vi "set_tilt_stage (SubVI).vi"(2 "stop":bool, 3 "Tot Stage Arr":dbl[](array[numeric]), 4 "tilt stage config":T2) -> (0 "thetaZ error out":errorcluster, 1 "thetaY error out":errorcluster)   [LabVIEW 2016]
uses:
  C:/Users/UsphereLab/Documents/GitHub/Optlev/LabView Code/Tilt Stage/CmdLib.dll
  Tilt Stage/CmdLib.dll
panel:
  in  "Axis inputs 5":T1={"Relative Steps"=0, "Motor Number"=1, "Run?"=FALSE, "Filename"=path "position.lvm", "CmdLib In"=refnum, "Device Address In"=0, "DeviceKey In"=""}
  in  "Axis inputs 4":T1={"Relative Steps"=0, "Motor Number"=1, "Run?"=FALSE, "Filename"=path "position.lvm", "CmdLib In"=refnum, "Device Address In"=0, "DeviceKey In"=""}
  in  "B Inputs":T1={"Relative Steps"=0, "Motor Number"=1, "Run?"=FALSE, "Filename"=path "position.lvm", "CmdLib In"=refnum, "Device Address In"=0, "DeviceKey In"=""}
  in  "A inputs":T1={"Relative Steps"=0, "Motor Number"=1, "Run?"=FALSE, "Filename"=path "position.lvm", "CmdLib In"=refnum, "Device Address In"=0, "DeviceKey In"=""}
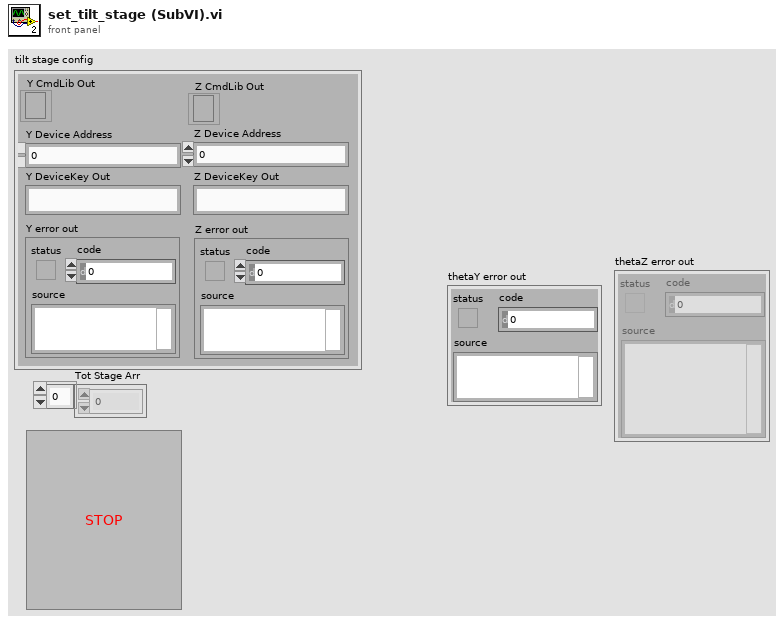
[diagram p1: front panel]
types:
  T1 = cluster{"Relative Steps":i32, "Motor Number":i32, "Run?":bool, "Filename":path, "CmdLib In":refnum<k24>, "Device Address In":i32, "DeviceKey In":string}
  T2 = cluster{"Y error out":errorcluster, "Y CmdLib Out":refnum<k24>, "Y Device Address":i32, "Y DeviceKey Out":string, "Z error out":errorcluster, "Z CmdLib Out":refnum<k24>, "Z Device Address":i32, "Z DeviceKey Out":string}
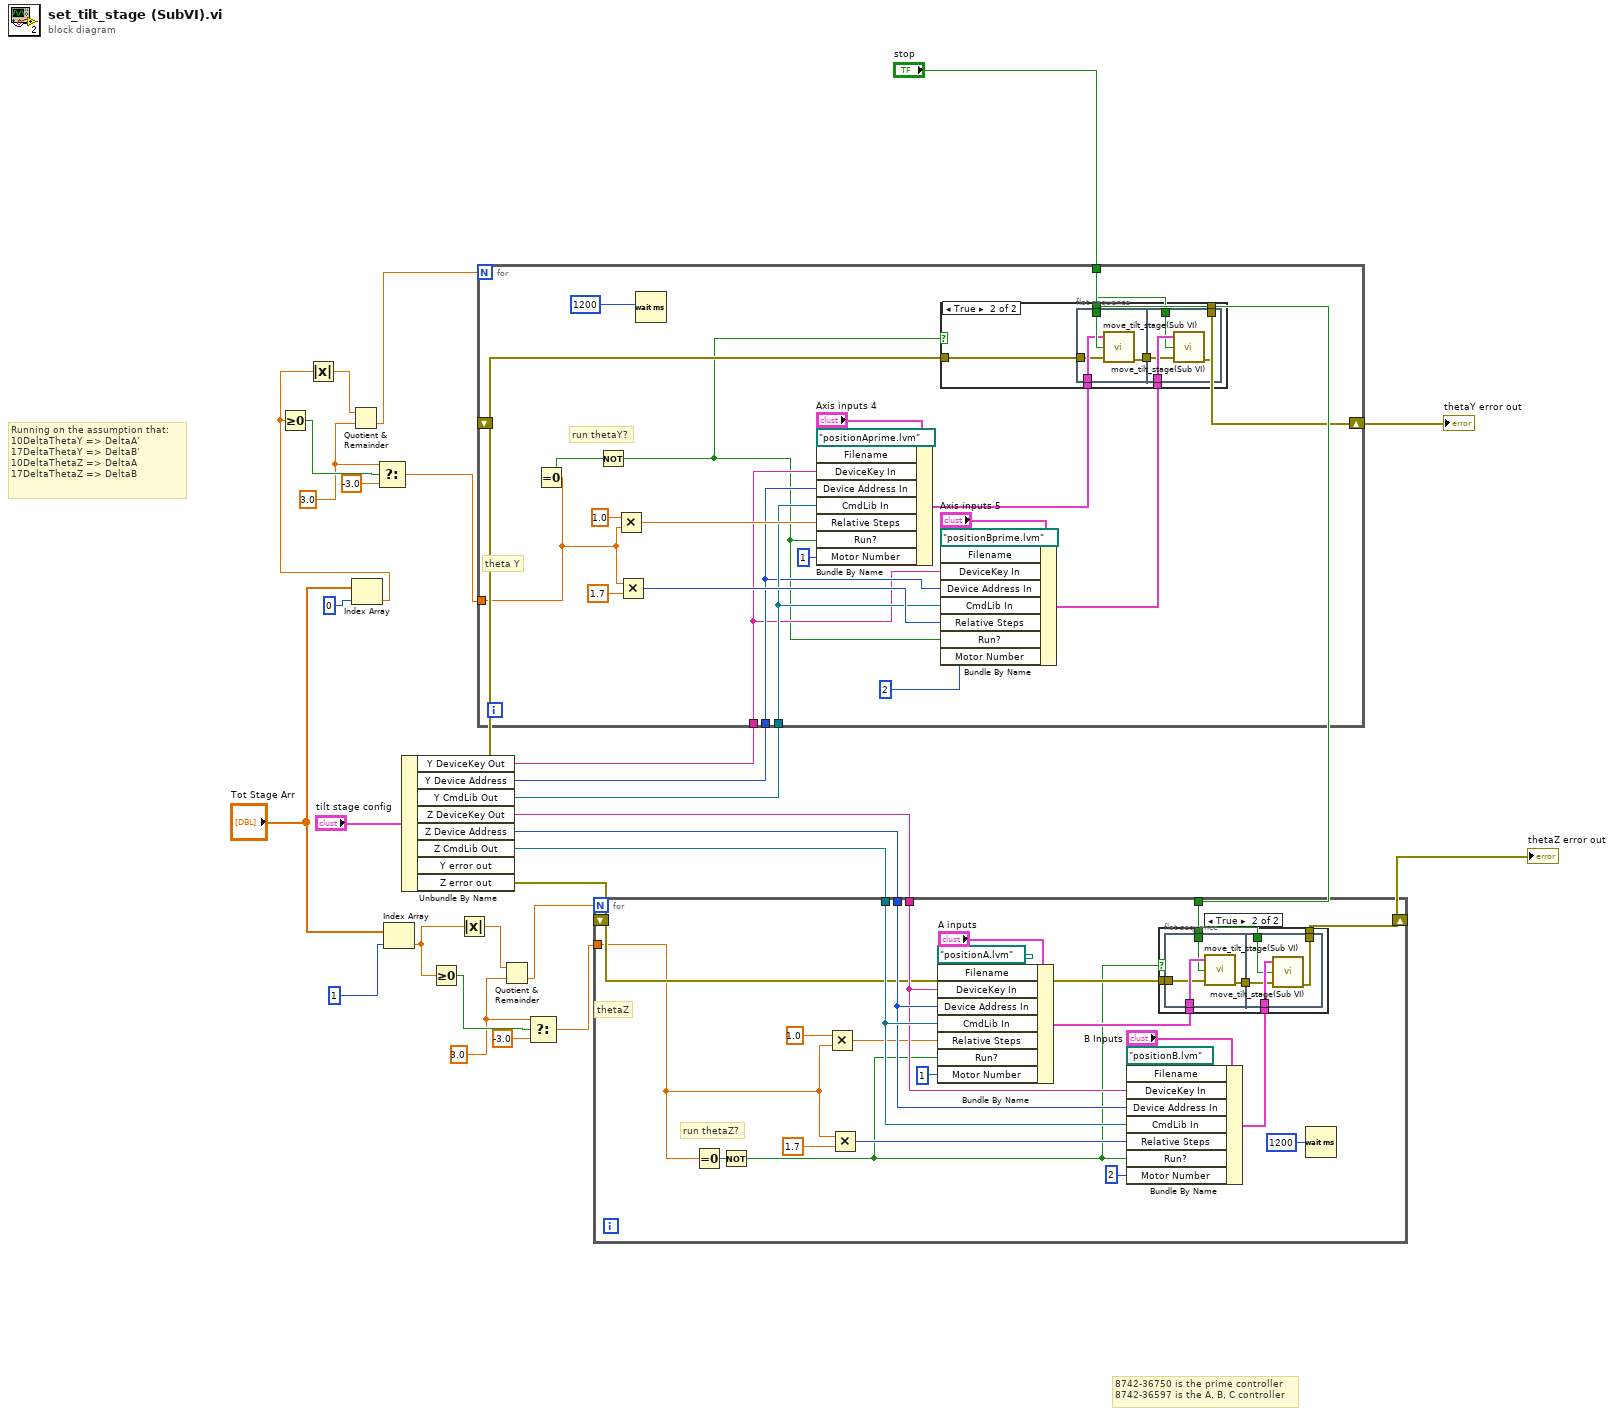
[diagram p0: block diagram]
diagram:
  w5 = 3.0 ("y")
  w10 = 3.0 ("y")
  # "Running on the assumption that:\n10DeltaThetaY => DeltaA'\n17DeltaThetaY => DeltaB'\n10DeltaThetaZ => DeltaA\n17DeltaThetaZ => DeltaB"
  # "8742-36750 is the prime controller\n8742-36597 is the A, B, C controller"
  n1 = Index Array(array="Tot Stage Arr", index=0 ("index (row)")) -> (element=w3:dbl)
  n2 = Greater Or Equal To 0?(x=w3) -> (x >= 0?=w6:bool)
  n3 = Absolute Value(x=w3) -> (abs(x)=w7:dbl)
  n4 = Quotient & Remainder(x=w7, y=w5) -> (floor(x/y)=w2:dbl)  [unwired: 1 out]
  n5 = Select(t=w5, s=w6, f=-3.0) -> (s? t:f=w1:dbl)
  n6 = Index Array(array="Tot Stage Arr", index=1 ("index (row)")) -> (element=w12:dbl)
  n7 = Unbundle By Name("tilt stage config") -> ("Y DeviceKey Out"=w18:string, "Y Device Address"=w19:i32, "Y CmdLib Out"=w20:refnum<k24>, "Z DeviceKey Out"=w21:string, "Z Device Address"=w22:i32, "Z CmdLib Out"=w23:refnum<k24>, "Y error out"=w24:errorcluster, "Z error out"=w15:errorcluster)
  n8 = Greater Or Equal To 0?(x=w12) -> (x >= 0?=w11:bool)
  n9 = Absolute Value(x=w12) -> (abs(x)=w13:dbl)
  n10 = for {
    N: w2 -> [_]
    tunnel: w20 -> [w37]
    tunnel: w19 -> [w36]
    tunnel: w18 -> [w35]
    tunnel: "stop" -> [w34]
    tunnel: w1 -> [w33]
    shift-right: [w43] -> w25
    shift-left: w24 -> [w40]
    # "run thetaY?"
    # "theta Y"
    n11 = Equal To 0?(x=w33) -> (x = 0?=w31:bool)
    n12 = Not(x=w31) -> (.not. x?=w32:bool)
    n13 = Multiply(x=1.0 ("10"), y=w33) -> (x*y=w42:dbl)
    n14 = Multiply(x=w33, y=1.7 ("17")) -> (x*y=w41:i16)
    n15 = Wait (ms)(milliseconds to wait=u32 1200) -> ()  [unwired: 1 out]
    n16 = Bundle By Name(cluster="Axis inputs 4", "Filename"=path "positionAprime.lvm", "DeviceKey In"=w35, "Device Address In"=w36, "CmdLib In"=w37, "Relative Steps"=w42, "Run?"=w32, "Motor Number"=1) -> (w39:T1)
    n17 = Bundle By Name(cluster="Axis inputs 5", "Filename"=path "positionBprime.lvm", "DeviceKey In"=w35, "Device Address In"=w36, "CmdLib In"=w37, "Relative Steps"=w41, "Run?"=w32, "Motor Number"=2) -> (w38:T1)
    n18 = case shown="True" w32 {
      tunnel: [w52 w57] -> w43
      tunnel: w40 -> [w52 w56]
      tunnel: w39 -> [_ w55]
      tunnel: w38 -> [_ w54]
      tunnel: w34 -> [_ w53]
      frame False {
      }
      frame True {
        n19 = flat-sequence {
          tunnel: w53 -> [w62]
          tunnel: w55 -> [w61]
          tunnel: [w60] -> w58
          tunnel: w56 -> [w59]
          tunnel: w54 -> [w66]
          tunnel: w53 -> [w65]
          tunnel: w58 -> [w64]
          tunnel: [w63] -> w57
          frame #0 {
            n20 = call "move_tilt_stage(Sub VI).vi"("Axis inputs"=w61, "stop"=w62, "error in (no error)"=w59) -> ("error out"=w60:errorcluster)  [unwired: 3 out]
          }
          frame #1 {
            n21 = call "move_tilt_stage(Sub VI).vi"("Axis inputs"=w66, "stop"=w65, "error in (no error)"=w64) -> ("error out"=w63:errorcluster)  [unwired: 3 out]
          }
        }
      }
    }
  }
  "thetaY error out" <- w25
  n22 = Quotient & Remainder(x=w13, y=w10) -> (floor(x/y)=w14:dbl)  [unwired: 1 out]
  n23 = Select(t=w10, s=w11, f=-3.0) -> (s? t:f=w8:dbl)
  n24 = for {
    N: w14 -> [_]
    tunnel: w23 -> [w80]
    tunnel: w22 -> [w79]
    tunnel: w21 -> [w78]
    tunnel: "stop" -> [w75]
    tunnel: w8 -> [w70]
    shift-right: [w74] -> w16
    shift-left: w15 -> [w71]
    # "run thetaZ?"
    # "thetaZ"
    n25 = Equal To 0?(x=w70) -> (x = 0?=w69:bool)
    n26 = Not(x=w69) -> (.not. x?=w68:bool)
    n27 = Multiply(x=1.0 ("10"), y=w70) -> (x*y=w77:dbl)
    n28 = Multiply(x=w70, y=1.7 ("17")) -> (x*y=w76:i16)
    n29 = Bundle By Name(cluster="A inputs", "Filename"=path "positionA.lvm", "DeviceKey In"=w78, "Device Address In"=w79, "CmdLib In"=w80, "Relative Steps"=w77, "Run?"=w68, "Motor Number"=1) -> (w72:T1)
    n30 = Bundle By Name(cluster="B Inputs", "Filename"=path "positionB.lvm", "DeviceKey In"=w78, "Device Address In"=w79, "CmdLib In"=w80, "Relative Steps"=w76, "Run?"=w68, "Motor Number"=2) -> (w73:T1)
    n31 = case shown="True" w68 {
      tunnel: w75 -> [_ w94]
      tunnel: [w89 w93] -> w74
      tunnel: w73 -> [_ w92]
      tunnel: w72 -> [_ w91]
      tunnel: w71 -> [w89 w90]
      frame False {
      }
      frame True {
        n32 = flat-sequence {
          tunnel: w91 -> [w99]
          tunnel: w94 -> [w98]
          tunnel: [w97] -> w95
          tunnel: w90 -> [w96]
          tunnel: w95 -> [w101]
          tunnel: w94 -> [w102]
          tunnel: w92 -> [w103]
          tunnel: [w100] -> w93
          frame #0 {
            n33 = call "move_tilt_stage(Sub VI).vi"("Axis inputs"=w99, "stop"=w98, "error in (no error)"=w96) -> ("error out"=w97:errorcluster)  [unwired: 3 out]
          }
          frame #1 {
            n34 = call "move_tilt_stage(Sub VI).vi"("Axis inputs"=w103, "stop"=w102, "error in (no error)"=w101) -> ("error out"=w100:errorcluster)  [unwired: 3 out]
          }
        }
      }
    }
    n35 = Wait (ms)(milliseconds to wait=u32 1200) -> ()  [unwired: 1 out]
  }
  "thetaZ error out" <- w16
